vi "SysLogHistory Dateien lesen.vi"(7 "Cluster PC cRIO History File":T1, 8 "Fehler (in)":errorcluster caption="Fehlerkonstante", 11 "Ebene":enum16{"PC+cRIO", "PC", "cRIO"}(ring)) -> (0 "Fehler (out)":errorcluster caption="Fehlerkonstante", 3 "Array-Typ (2D Dbl)":string[][](array[string]))   [LabVIEW 2015, in "SysLog.lvlib"]
uses:
  SysLog.lvlib
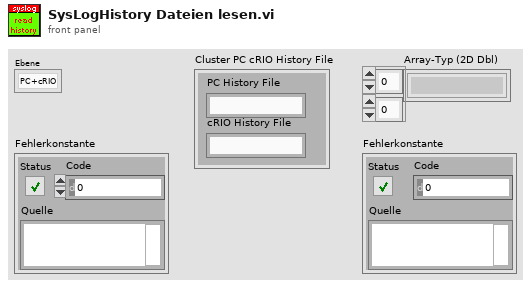
[diagram p1: front panel]
types:
  T1 = cluster{"PC History File":string, "cRIO History File":string}
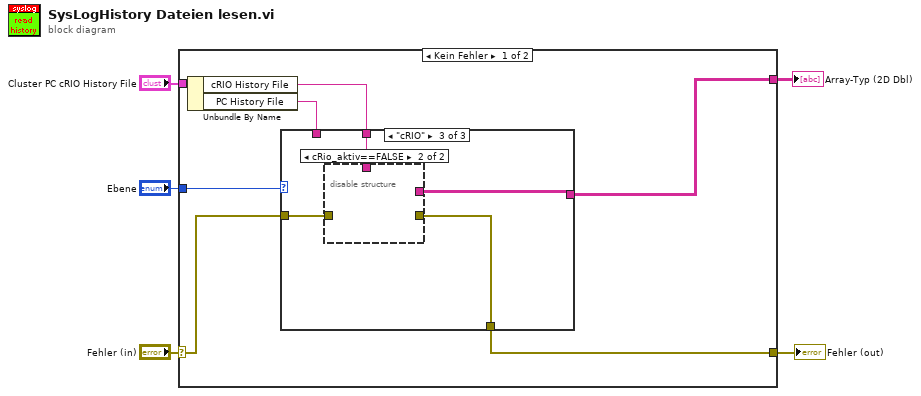
[diagram p0: block diagram]
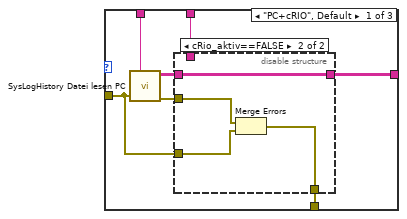
[diagram p2: hidden frame]
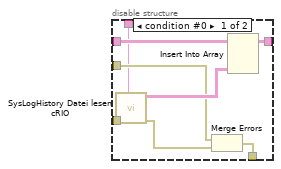
[diagram p3: hidden frame]
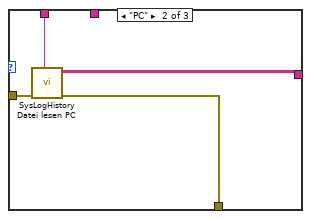
[diagram p4: hidden frame]
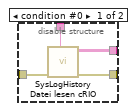
[diagram p5: hidden frame]
diagram:
  n1 = case shown="Kein Fehler" "Fehler (in)" {
    selector: "Fehler (in)" -> [w11 w44]
    tunnel: [w10 w44] -> w4
    tunnel: [w12 _] -> w3
    tunnel: "Ebene" -> [w9 _]
    tunnel: "Cluster PC cRIO History File" -> [w8 _]
    frame No Error {
      n2 = Unbundle By Name(w8) -> ("cRIO History File"=w6:string, "PC History File"=w7:string)
      n3 = case shown="\"cRIO\"" w9 {
        tunnel: [w19 w34 w38] -> w12
        tunnel: w11 -> [w17 w35 w39]
        tunnel: [w16 w33 w37] -> w10
        tunnel: w7 -> [w14 w32 _]
        tunnel: w6 -> [w13 _ w36]
        frame "PC+cRIO", Default {
          n4 = call "SysLogHistory Datei lesen PC.vi"("History File"=w14, "Fehler (in)"=w17) -> ("Fehler (out)"=w15:errorcluster, "Array-Typ (2D Dbl)"=w18:string[][])  [unwired: 8 in]
          n5 = disable-structure shown="cRio_aktiv==FALSE" {
            disable-tunnel: [w27 w31] -> w19
            disable-tunnel: w18 -> [w26 w31]
            disable-tunnel: w17 -> [w24 w29]
            disable-tunnel: [w23 w28] -> w16
            disable-tunnel: w15 -> [w22 w30]
            disable-tunnel: w13 -> [w20 _]
            frame condition #0 {
              n6 = call "SysLogHistory Datei lesen cRIO.vi"("History File"=w20, "Fehler (in)"=w24) -> ("Fehler (out)"=w21:errorcluster, "Array-Typ (2D Dbl)"=w25:string[][])  [unwired: 8 in]
              n7 = Merge Errors(w22, w21) -> (w23:errorcluster)
              n8 = Insert Into Array(array=w26, new element=w25) -> (w27:string[][])  [unwired: 2 in]
            }
            frame condition #1 (active) {
              n9 = Merge Errors(w30, w29) -> (w28:errorcluster)
            }
          }
        }
        frame "PC" {
          n10 = call "SysLogHistory Datei lesen PC.vi"("History File"=w32, "Fehler (in)"=w35) -> ("Fehler (out)"=w33:errorcluster, "Array-Typ (2D Dbl)"=w34:string[][])  [unwired: 8 in]
        }
        frame "cRIO" {
          n11 = disable-structure shown="cRio_aktiv==FALSE" {
            disable-tunnel: w39 -> [w43 _]
            disable-tunnel: [w42 _] -> w38
            disable-tunnel: [w41 _] -> w37
            disable-tunnel: w36 -> [w40 _]
            frame condition #0 {
              n12 = call "SysLogHistory Datei lesen cRIO.vi"("History File"=w40, "Fehler (in)"=w43) -> ("Fehler (out)"=w41:errorcluster, "Array-Typ (2D Dbl)"=w42:string[][])  [unwired: 8 in]
            }
            frame condition #1 (active) {
            }
          }
        }
      }
    }
    frame Error {
    }
  }
  "Fehler (out)" <- w4
  "Array-Typ (2D Dbl)" <- w3
